vi "Initialize_w_RS232.vi"(8 "error in (no error)":errorcluster, 9 "Reset (True)":bool=TRUE, 10 "ID Query (True)":bool=TRUE, 11 "VISA resource name":refnum<visa-resource-name>) -> (0 "error out":errorcluster, 3 "VISA resource name out":refnum<visa-resource-name>)   [LabVIEW 2015, in "Keithley DMM6500 DAQ6500 Series.lvlib"]
doc: "Establishes communication with the instrument and optionally performs an instrument identification query and/or an instrument reset. It also places the instrument in a default state needed for other instrument driver operations. Therefore, call this VI before calling other instrument driver VIs for this instrument. Generally, you need to call the <b>Initialize</b> VI only once at the beginning of an application."
uses:
  <instrlib>/Keithley DMM6500 DAQ6500 Series/Keithley DMM6500 DAQ6500 Series.lvlib
panel:
  # "(c) 2018 National Instruments.  ALL RIGHTS RESERVED."
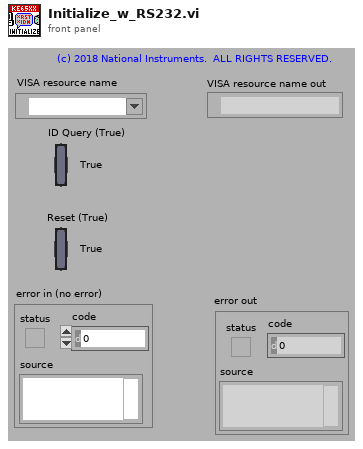
[diagram p1: front panel]
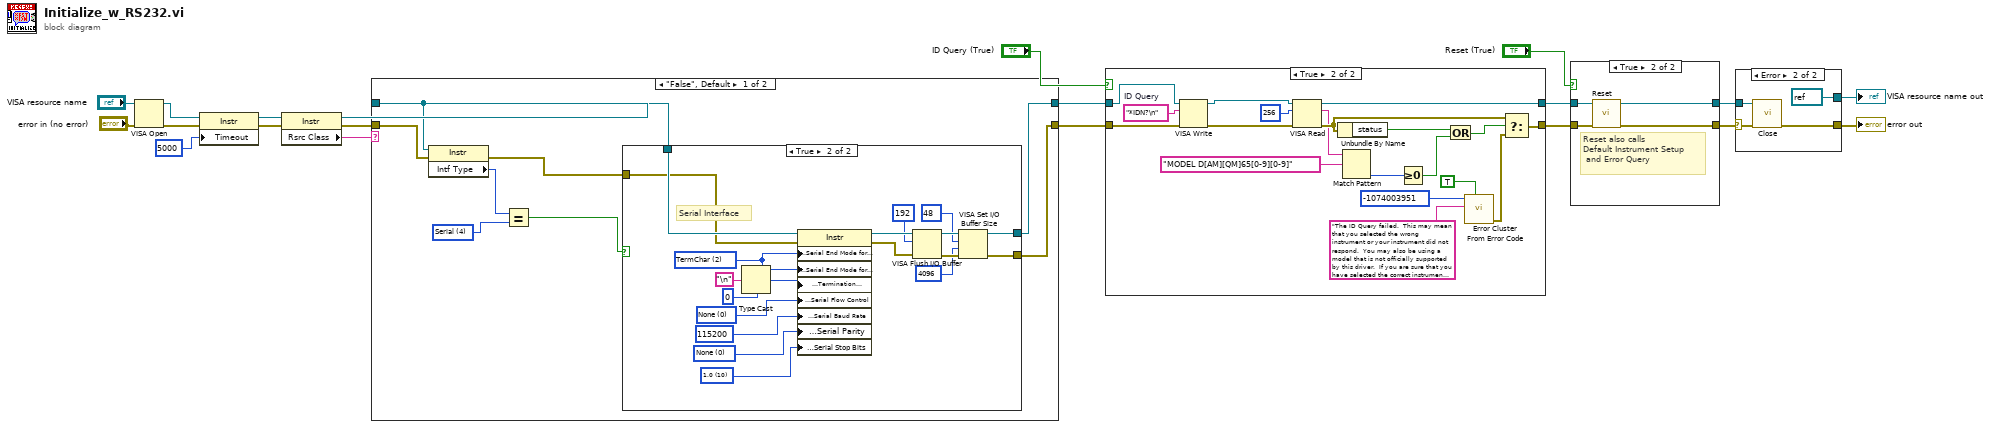
[diagram p0: block diagram]
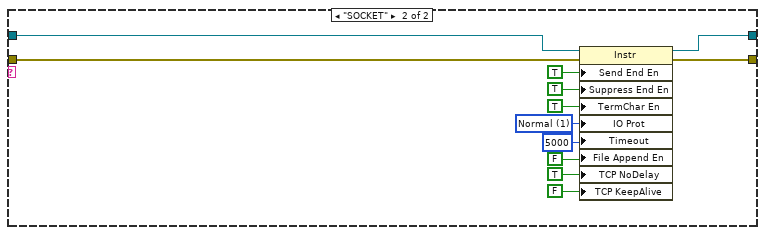
[diagram p3: hidden frame]
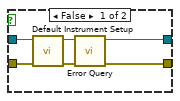
[diagram p5: hidden frame]
diagram:
  n1 = VISA Open(error in (no error)="error in (no error)", VISA resource name="VISA resource name") -> (VISA resource name=w4:refnum<visa-resource-name>, error out=w3:errorcluster)  [unwired: 3 in]
  n2 = property class="Instr"(reference=w4, error in=w3, "Timeout"=u32 5000 ("General Settings:Timeout Value")) -> (reference out=w1:refnum<visa-resource-name>, error out=w2:errorcluster)
  n3 = property class="Instr"(reference=w1, error in=w2) -> (reference out=w9:refnum<visa-resource-name>, error out=w8:errorcluster, "Rsrc Class"=w10:string)
  n4 = case shown="\"False\", Default" w10 {
    tunnel: w9 -> [w28 w58]
    tunnel: w8 -> [w27 w57]
    tunnel: [w25 w60] -> w7
    tunnel: [w24 w59] -> w6
    frame "False", Default {
      w22 = u16 4 items=["GPIB"=1, "VXI"=2, "GPIB-VXI"=3, "Serial"=4, "PXI"=5, "TCPIP"=6, "USB"=7, "FireWire"=9] ("Interface Information:Interface Type")
      n5 = property class="Instr"(reference=w28, error in=w27) -> (error out=w26:errorcluster, "Intf Type"=w23:u16)  [unwired: 1 out]
      n6 = Equal?(x=w23, y=w22) -> (x = y?=w21:bool)
      n7 = case shown="True" w21 {
        tunnel: w28 -> [w29 w34]
        tunnel: w26 -> [w30 w33]
        tunnel: [w29 w32] -> w25
        tunnel: [w30 w31] -> w24
        frame False {
        }
        frame True {
          w35 = u16 10 items=["1.0"=10, "1.5"=15, "2.0"=20] ("Serial Settings:Serial Stop Bits")
          w38 = u16 0 items=["None", "Odd", "Even", "Mark", "Space"] ("Serial Settings:Serial Parity")
          w40 = u16 2 items=["None", "LastBit", "TermChar"] ("Serial Settings:Serial End Mode for Reads")
          w36 = u16 0 items=["None"=0, "XON/XOFF"=1, "RTS/CTS"=2, "DTR/DSR"=4] ("Serial Settings:Serial Flow Control")
          # "Serial Interface"
          n8 = Type Cast(type=u8 0, x="\n") -> (*(type *) &x=w39:u8)
          n9 = property class="Instr"(reference=w34, error in=w33, "Serial Settings:Serial End Mode for Reads"=w40, "Serial Settings:Serial End Mode for Writes"=w40, "Message Based Settings:Termination Character"=w39, "Serial Settings:Serial Flow Control"=w36, "Serial Settings:Serial Baud Rate"=u32 115200, "Serial Settings:Serial Parity"=w38, "Serial Settings:Serial Stop Bits"=w35) -> (reference out=w46:refnum<visa-resource-name>, error out=w48:errorcluster)
          n10 = VISA Flush I/O Buffer(VISA resource name=w46, mask (16)=u16 192, error in (no error)=w48) -> (VISA resource name out=w49:refnum<visa-resource-name>, error out=w47:errorcluster)
          n11 = VISA Set I/O Buffer Size(VISA resource name=w49, mask (16)=u16 48, size (4096)=u32 4096 ("size (0)"), error in (no error)=w47) -> (VISA resource name out=w32:refnum<visa-resource-name>, error out=w31:errorcluster)
        }
      }
    }
    frame "SOCKET" {
      w53 = u16 1 items=["Normal"=1, "VXI/FDC"=2, "GPIB/HS488"=3, "Serial-TCPIP-USB/488 Strings"=4, "USBTMC/Vendor-Specific"=5] ("Message Based Settings:IO Protocol")
      n12 = property class="Instr"(reference=w58, error in=w57, "Send End En"=TRUE ("Message Based Settings:Termination Character Enable"), "Suppress End En"=TRUE ("Message Based Settings:Suppress End Enable"), "TermChar En"=TRUE ("Message Based Settings:Termination Character Enable"), "IO Prot"=w53, "Timeout"=u32 5000 ("General Settings:Timeout Value"), "File Append En"=FALSE ("Message Based Settings:File Append Enable"), "TCP NoDelay"=TRUE ("TCP/IP Settings:No Packet Delay"), "TCP KeepAlive"=FALSE ("TCP/IP Settings:Keep-Alive Packets")) -> (reference out=w60:refnum<visa-resource-name>, error out=w59:errorcluster)
    }
  }
  n13 = case shown="True" "ID Query (True)" {
    tunnel: [w62 w82] -> w19
    tunnel: [w63 w81] -> w20
    tunnel: w7 -> [w63 w65]
    tunnel: w6 -> [w62 w64]
    frame False {
    }
    frame True {
      w76 = "*IDN?\n"  # ID Query
      n14 = VISA Write(VISA resource name=w65, write buffer=w76, error in (no error)=w64) -> (VISA resource name out=w80:refnum<visa-resource-name>, error out=w79:errorcluster)  [unwired: 1 out]
      n15 = VISA Read(VISA resource name=w80, byte count=u32 256, error in (no error)=w79) -> (VISA resource name out=w81:refnum<visa-resource-name>, read buffer=w66:string, error out=w70:errorcluster)  [unwired: 1 out]
      n16 = Unbundle By Name(w70) -> ("status"=w69:bool)
      n17 = Match Pattern(string=w66, regular expression="MODEL D[AM][QM]65[0-9][0-9]") -> (offset past match=w71:i32)  [unwired: 1 in, 3 out]
      n18 = Greater Or Equal To 0?(x=w71) -> (x >= 0?=w68:bool)
      n19 = Or(x=w69, y=w68) -> (x .or. y?=w67:bool)
      n20 = call <vilib>:"Error Cluster From Error Code.vi"("show call chain? (False)"=TRUE, "error message (\"\")"="The ID Query failed.  This may mean that you selected the wrong instrument or your instrument did not respond.  You may also be using a model that is not officially supported by this driver.  If you are sure that you have selected the correct instrument and it is responding, try disabling the ID Query." ("Source (VI Name)"), "error code (0)"=-1074003951 ("Code")) -> ("error out"=w75:errorcluster)  [unwired: 6 in]
      n21 = Select(t=w70, s=w67, f=w75) -> (s? t:f=w82:errorcluster)
    }
  }
  n22 = case shown="True" "Reset (True)" {
    tunnel: w19 -> [w87 w89]
    tunnel: [w84 w92] -> w11
    tunnel: w20 -> [w88 w90]
    tunnel: [w85 w91] -> w12
    frame False {
      n23 = call <instrlib>:"Default Instrument Setup.vi"("error in (no error)"=w87, "VISA resource name"=w88) -> ("error out"=w83:errorcluster, "VISA resource name out"=w86:refnum<visa-resource-name>)  [unwired: 8 in]
      n24 = call <instrlib>:"Error Query.vi"("error in (no error)"=w83, "VISA resource name"=w86) -> ("error out"=w84:errorcluster, "VISA resource name out"=w85:refnum<visa-resource-name>)  [unwired: 6 in, 2 out]
    }
    frame True {
      # "Reset also calls \nDefault Instrument Setup\n and Error Query"
      n25 = call <instrlib>:"Reset.vi"("error in (no error)"=w89, "VISA resource name"=w90) -> ("error out"=w92:errorcluster, "VISA resource name out"=w91:refnum<visa-resource-name>)  [unwired: 8 in]
    }
  }
  n26 = case shown="Error" w11 {
    selector: w11 -> [w93 w96]
    tunnel: w12 -> [w94 w97]
    tunnel: [w94 refnum<visa-resource-name> refnum ("VISA resource name out")] -> w14
    tunnel: [w93 w98] -> w13
    frame No Error {
    }
    frame Error {
      n27 = call <instrlib>:"Close.vi"("error in (no error)"=w96, "VISA resource name"=w97) -> ("error out"=w98:errorcluster)  [unwired: 9 in]
    }
  }
  "VISA resource name out" <- w14
  "error out" <- w13
